vi "CoffeeVending.vi"() -> ()   [LabVIEW 2020, in "CoffeeVending.lvlib"]
uses:
  CoffeeVending.lvlib
  TypeDef/QOperation.ctl
  TypeDef/CoffeeVendingCluster.ctl
  <vilib>/Utility/config.llb/Config Data RefNum.ctl
  <vilib>/Utility/config.llb/Read Key (I32).vi
  <vilib>/Utility/config.llb/Read Key (Boolean).vi
  <vilib>/Utility/config.llb/NI_LVConfig.lvlib
panel:
  in  "Power":bool
  out "Total Cups":i32
  out "Elapsed Time":i32
  out "Dispensing":bool
  out "Brewing":bool
  out "Grinding":bool
  out "Heating":bool
  out "Purging":bool
  out "Low Milk":bool
  out "Low Bean":bool
  out "Low Water":bool
  out "Dispenser":dbl(slide) scale=0.0..60.0
  out "Chamber":dbl(slide) scale=0.0..60.0
  in  "Milk Level":dbl(slide) scale=0.0..100.0
  in  "Bean Level":dbl(slide) scale=0.0..100.0
  in  "Water Level":dbl(slide) scale=0.0..100.0
  in  "Vending Type":i32(knob) scale=0.0..2.0
  in  "Carafe":bool
  in  "Cup":bool
  in  "error in":errorcluster
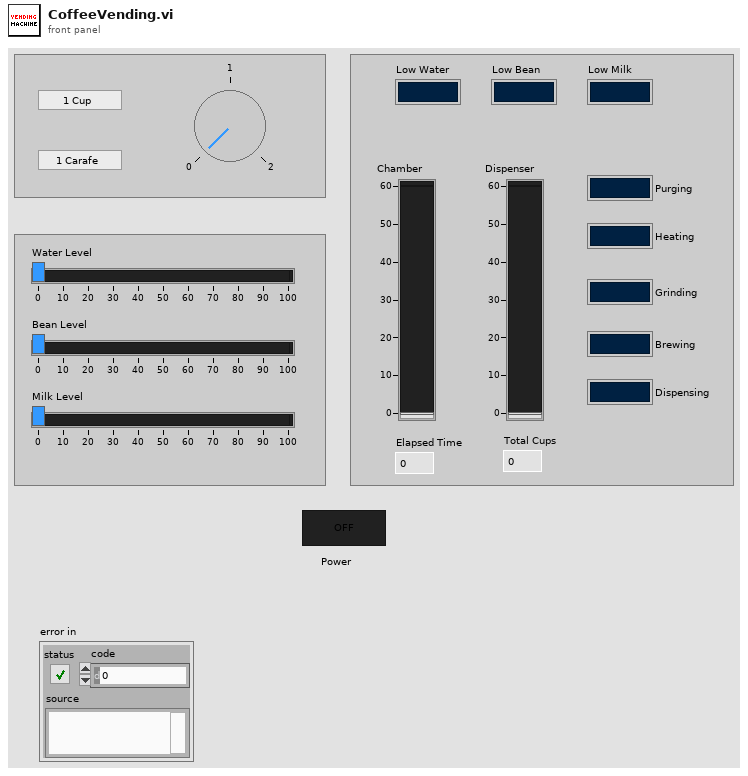
[diagram p1: front panel]
types:
  T1 = typedef "CoffeeVending.lvlib/CoffeeVendingCluster.ctl" = cluster{"Carafe":bool, "Cup":bool, "Water Level":dbl, "Bean Level":dbl, "Milk Level":dbl, "Low Milk":bool, "Low Bean":bool, "Low Water":bool, "Dispenser":dbl, "Chamber":dbl, "Purging":bool, "Brewing":bool, "Heating":bool, "Grinding":bool, "Dispensing":bool, "Elapsed Time":i32, "Total Cups":i32, "File Path":path, "File Reference":T2, "Power":bool, "Start Time":dbl, "Duration":dbl, "Sequence":string[], "Index":i32, "Flag":i32, "Latte":bool}
  T2 = typedef "NI_LVConfig.lvlib/Config Data RefNum.ctl" = refnum<k1>
  T3 = typedef "CoffeeVending.lvlib/QOperation.ctl" = enum16{"Init", "Enqueue", "Dequeue", "Enqueue N", "Enstack", "Release", "Flush"}
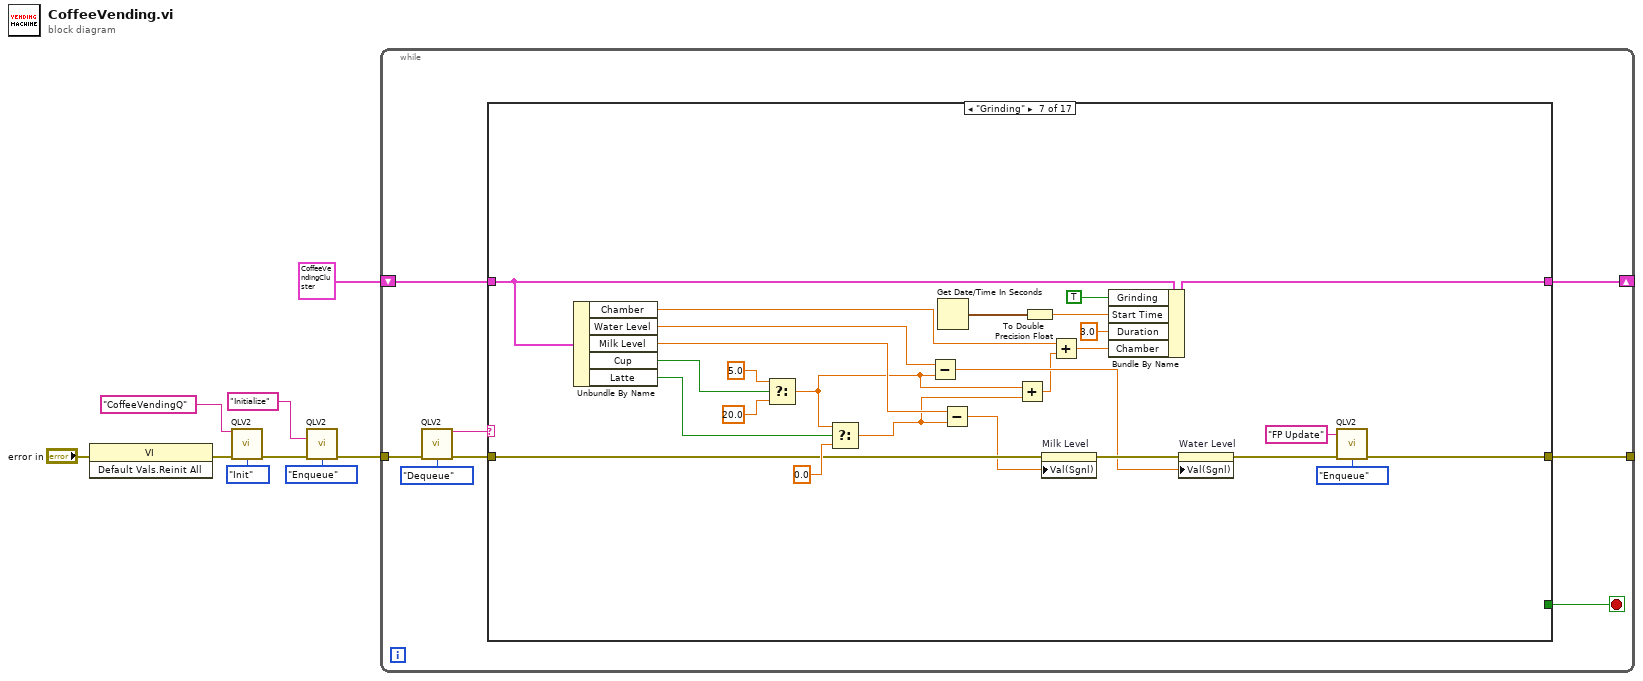
[diagram p0: block diagram]
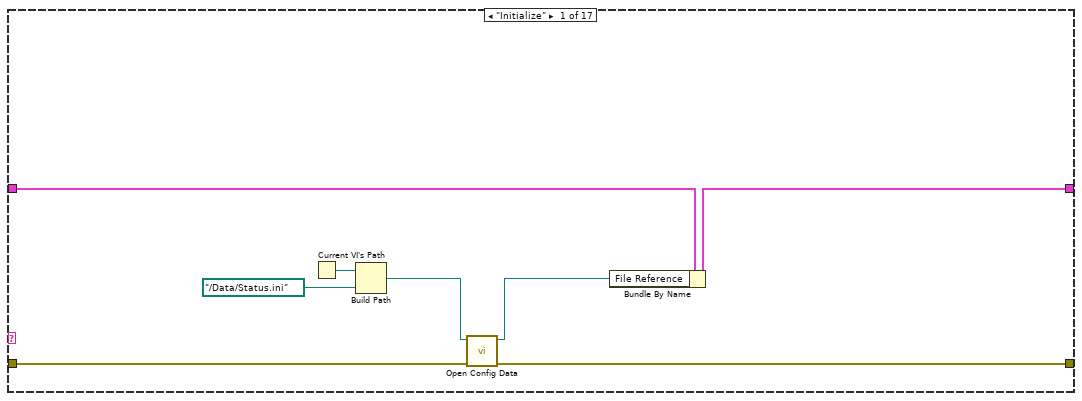
[diagram p2: hidden frame]
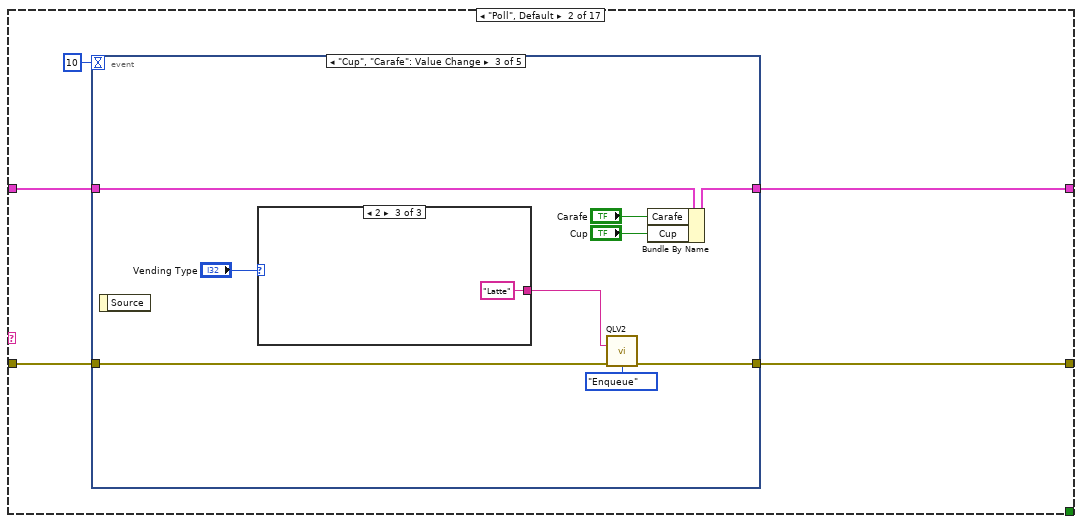
[diagram p3: hidden frame]
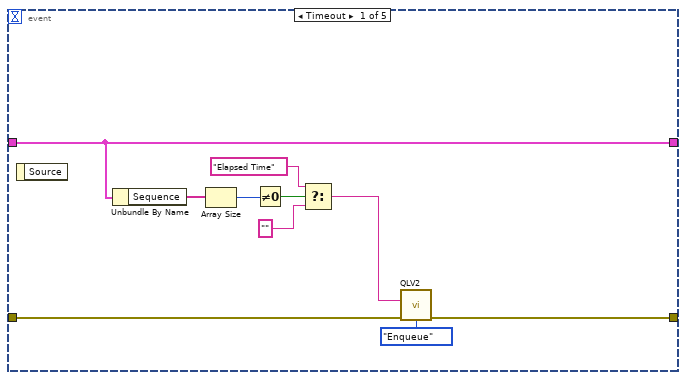
[diagram p4: hidden frame]
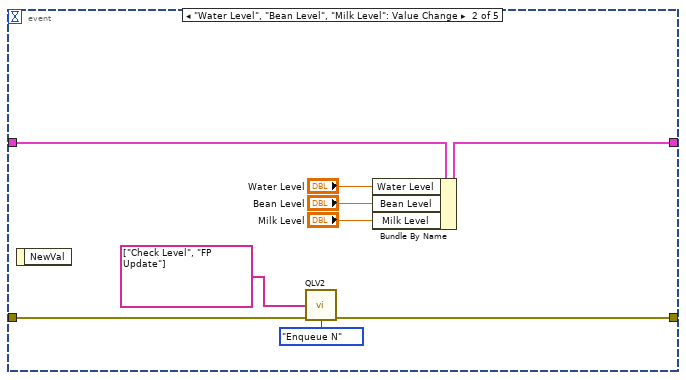
[diagram p5: hidden frame]
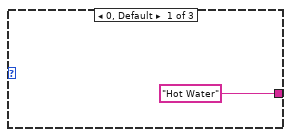
[diagram p6: hidden frame]
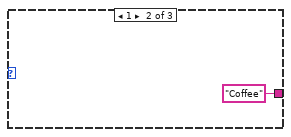
[diagram p7: hidden frame]
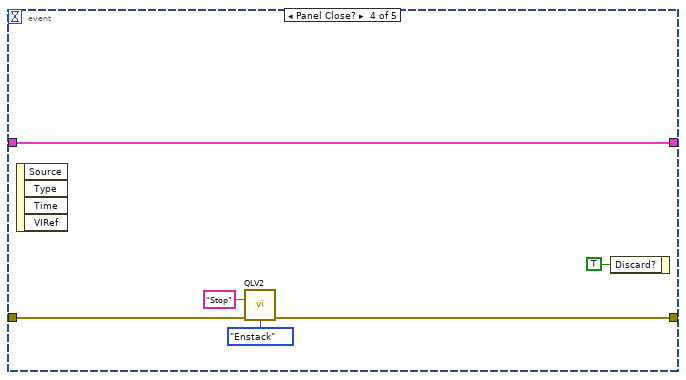
[diagram p8: hidden frame]
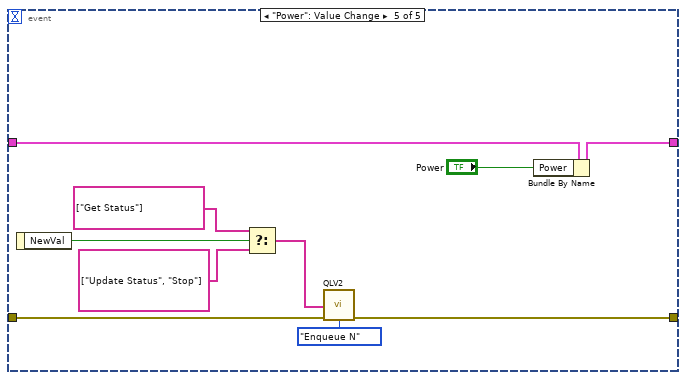
[diagram p9: hidden frame]
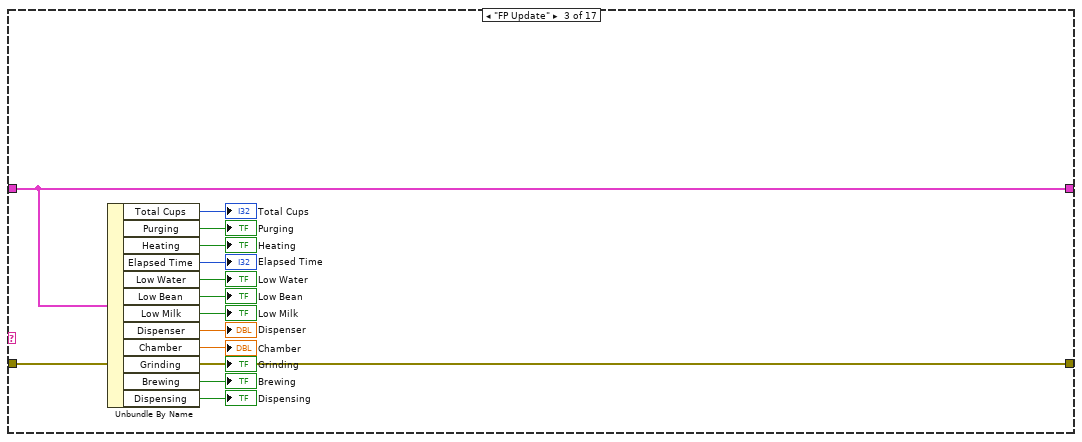
[diagram p10: hidden frame]
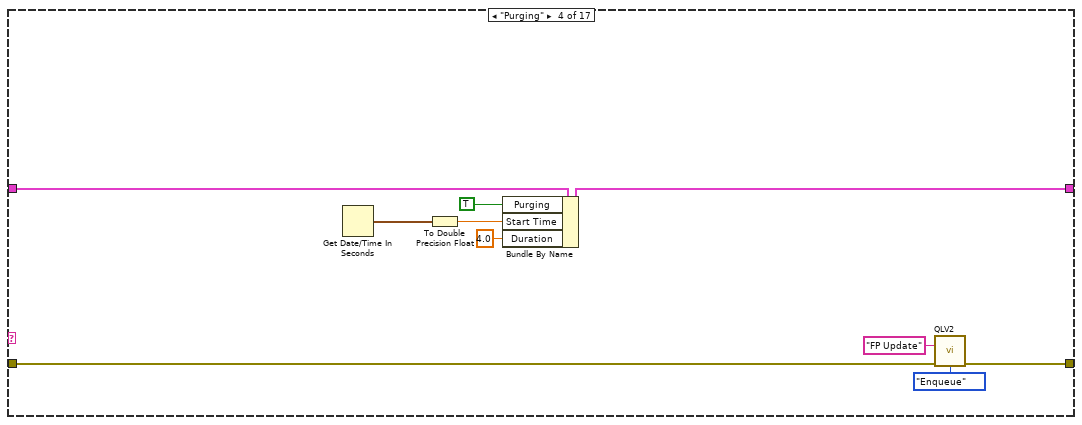
[diagram p11: hidden frame]
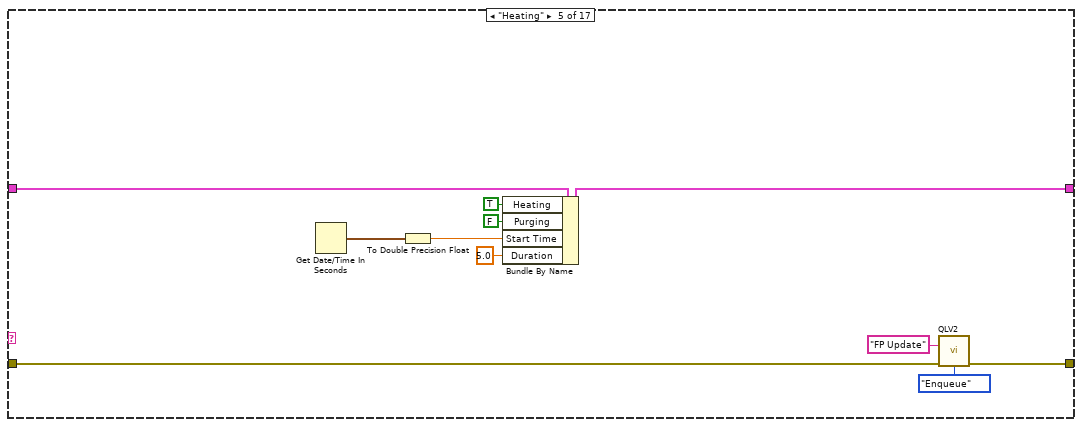
[diagram p12: hidden frame]
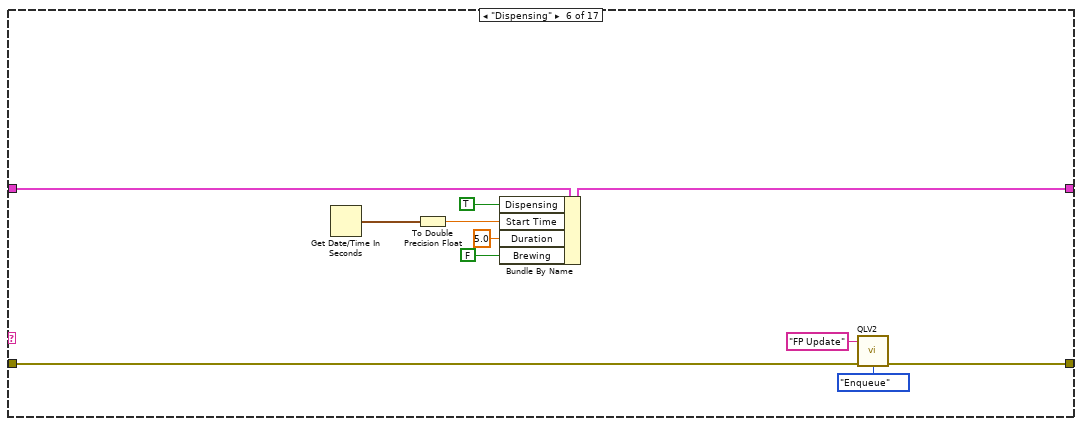
[diagram p13: hidden frame]
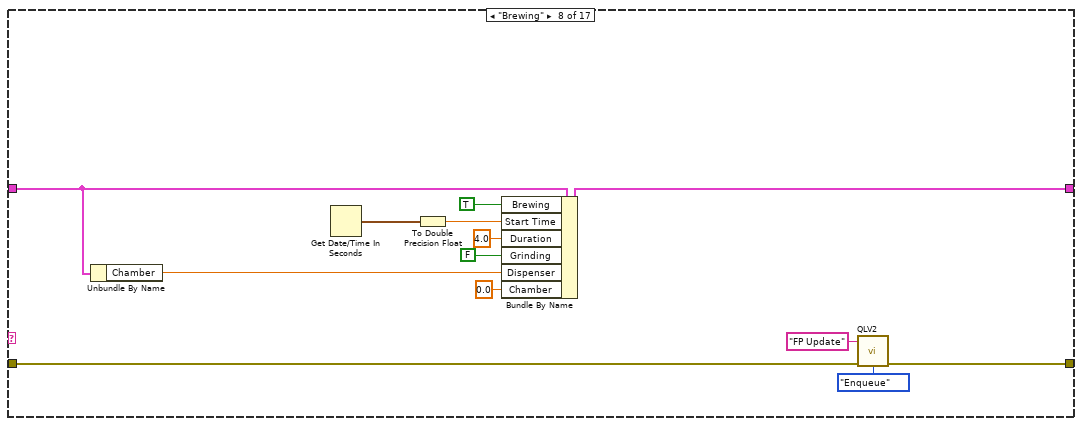
[diagram p14: hidden frame]
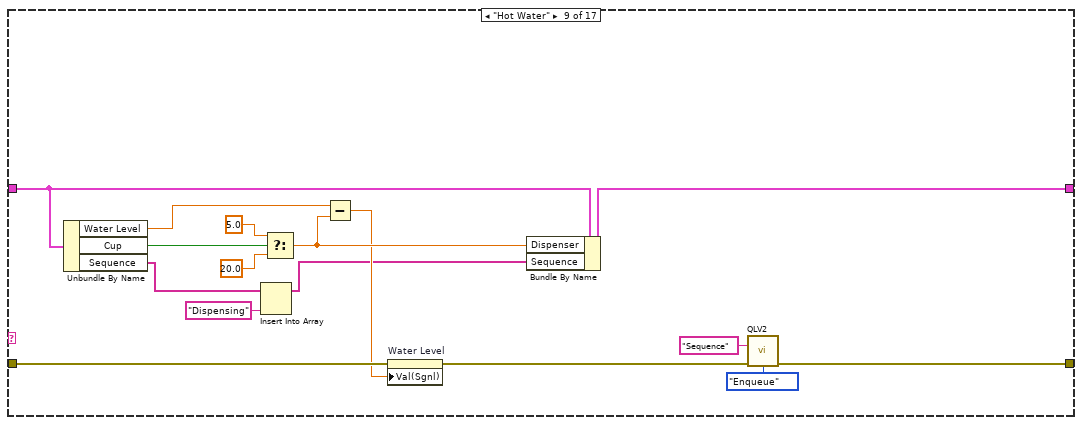
[diagram p15: hidden frame]
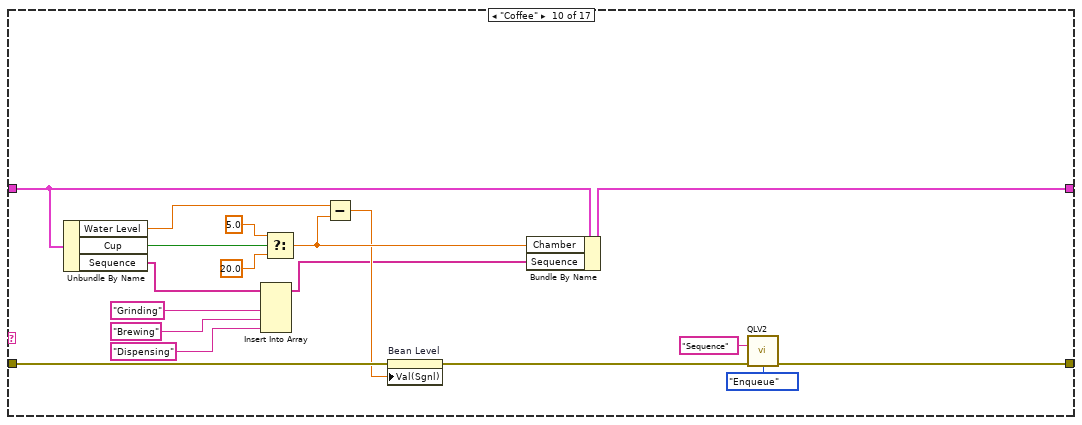
[diagram p16: hidden frame]
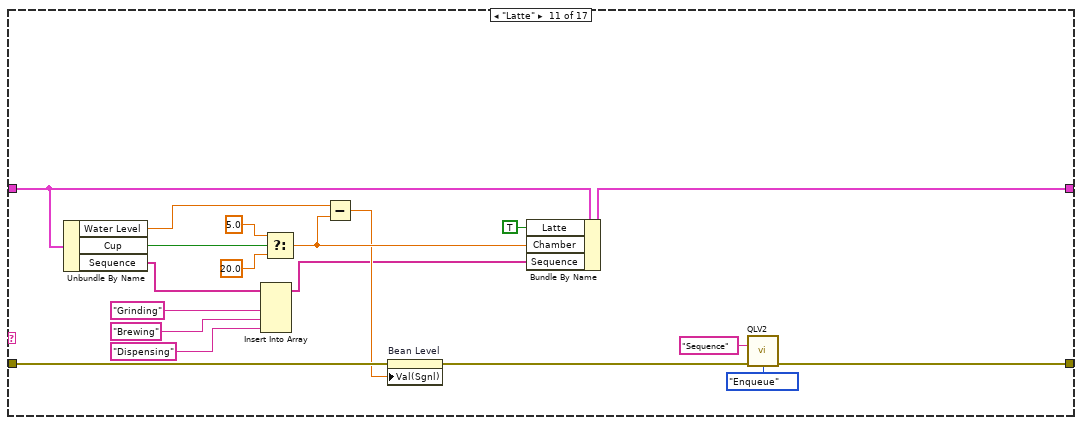
[diagram p17: hidden frame]
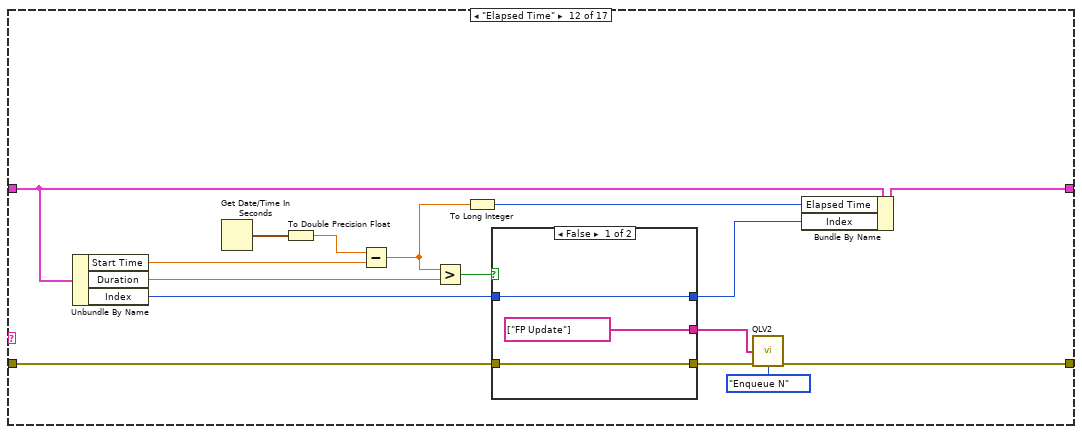
[diagram p18: hidden frame]
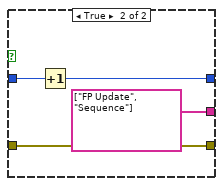
[diagram p19: hidden frame]
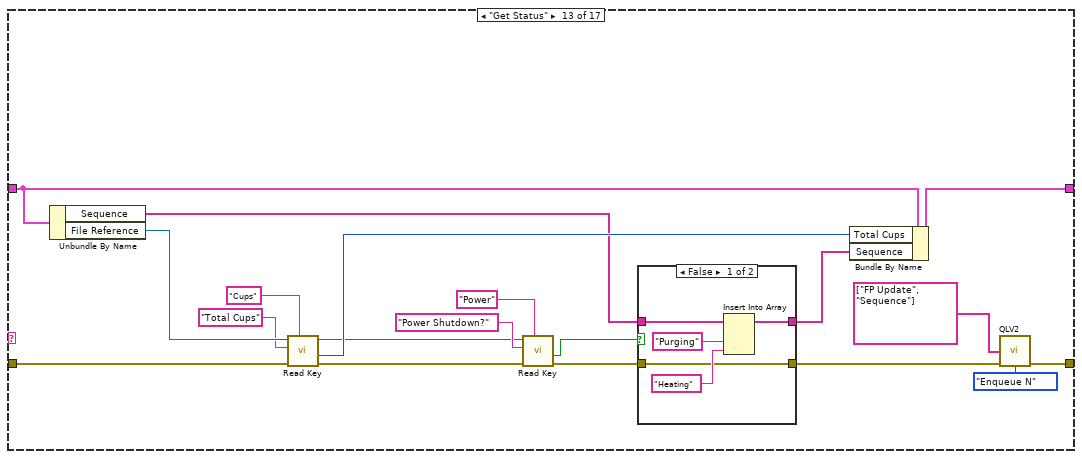
[diagram p20: hidden frame]
diagram:
  n1 = invoke class="VI" method="Default Vals.Reinit All"(error in="error in") -> (error out=w8:errorcluster)  [unwired: 2 in, 2 out]
  n2 = call "QLV2.vi"("Name"="CoffeeVendingQ", "error in"=w8, "Operation"=QOperation."Init") -> ("error out"=w5:errorcluster)  [unwired: 11 in, 1 out]
  n3 = call "QLV2.vi"("States"="Initialize", "error in"=w5, "Operation"=QOperation."Enqueue") -> ("error out"=w2:errorcluster)  [unwired: 11 in, 1 out]
  n4 = while {
    tunnel: w2 -> [w17]
    shift-right: [w12] -> _
    shift-left: T1 {"Carafe"=FALSE, "Cup"=FALSE, "Water Level"=0.0, "Bean Level"=0.0, "Milk Level"=0.0, "Low Milk"=FALSE, "Low Bean"=FALSE, "Low Water"=FALSE, "Dispenser"=0.0, "Chamber"=0.0, "Purging"=FALSE, "Brewing"=FALSE, "Heating"=FALSE, "Grinding"=FALSE, "Dispensing"=FALSE, "Elapsed Time"=0, "Total Cups"=0, "File Path"=path "", "File Reference"=refnum, "Power"=FALSE, "Start Time"=0.0, "Duration"=0.0, "Sequence"=[], "Index"=0, "Flag"=0, "Latte"=FALSE} -> [w13]
    tunnel: [w11] -> _
    stop <- w10 stop-if-true
    n5 = call "QLV2.vi"("error in"=w17, "Operation"=QOperation."Dequeue") -> ("State Out"=w15:string, "error out"=w14:errorcluster)  [unwired: 12 in]
    n6 = case shown="\"Grinding\"" w15 {
      tunnel: w14 -> [w18 w27 w89 w97 w106 w115 w132 w155 w173 w191 w210 w217 w256 w273 w308 w313 w326]
      tunnel: w13 -> [w25 w29 w90 w101 w112 w123 w141 w152 w175 w193 w212 w228 w251 w275 w303 w318 w329]
      tunnel: [w24 w28 w90 w100 w111 w122 w149 w162 w174 w192 w211 w227 w250 w274 w312 w317 w329] -> w12
      tunnel: [w21 w26 w89 w96 w105 w114 w142 w154 w164 w182 w201 w224 w248 w280 w307 w313 w323] -> w11
      tunnel: [_ _ _ _ _ _ _ _ _ _ _ _ _ _ _ _ TRUE] -> w10
      frame "Initialize" {
        n7 = Current VI's Path() -> (path=w23:path)
        n8 = Build Path(base path=w23, name or relative path=path "../Data/Status.ini") -> (appended path=w20:path)
        n9 = call <vilib>:"Open Config Data.vi"("error in (no error)"=w18, "configuration file path"=w20) -> ("error out"=w21:errorcluster, "refnum"=w19:T2)  [unwired: 7 in, 1 out]
        n10 = Bundle By Name(cluster=w25, "File Reference"=w19) -> (w24:T1)
      }
      frame "Poll", Default {
        n11 = event shown="[2] \"Cup\", \"Carafe\": Value Change" {
          selector: _ -> [_ _ _ _ _]
          dyn-events: _ -> [_ _ _ _ _]
          timeout: 10 -> [_ _ _ _ _]
          tunnel: w29 -> [w40 w49 w54 w62 w73]
          tunnel: [w40 w48 w52 w62 w72] -> w28
          tunnel: w27 -> [w33 w46 w56 w65 w76]
          tunnel: [w32 w45 w55 w64 w75] -> w26
          event Timeout {
            n12 = event-data() -> ()  [unwired: 1 in, 1 out]
            n13 = Unbundle By Name(w40) -> ("Sequence"=w39:string[])
            n14 = Array Size(array=w39) -> (size(s)=w38:i32)
            n15 = Not Equal To 0?(x=w38) -> (x != 0?=w37:bool)
            n16 = Select(t="Elapsed Time", s=w37, f="") -> (s? t:f=w31:string)
            n17 = call "QLV2.vi"("States"=w31, "error in"=w33, "Operation"=QOperation."Enqueue") -> ("error out"=w32:errorcluster)  [unwired: 11 in, 1 out]
          }
          event "Water Level", "Bean Level", "Milk Level": Value Change {
            n18 = event-data() -> ()  [unwired: 1 in, 1 out]
            n19 = call "QLV2.vi"("States[]"=string[] ["Check Level", "FP Update"], "error in"=w46, "Operation"=QOperation."Enqueue N") -> ("error out"=w45:errorcluster)  [unwired: 11 in, 1 out]
            n20 = Bundle By Name(cluster=w49, "Water Level"="Water Level", "Bean Level"="Bean Level", "Milk Level"="Milk Level") -> (w48:T1)
          }
          event "Cup", "Carafe": Value Change {
            n21 = event-data() -> ()  [unwired: 1 in, 1 out]
            n22 = case shown="2" "Vending Type" {
              tunnel: ["Hot Water" ("State Out") "Coffee" ("State Out") "Latte" ("State Out")] -> w53
              frame 0, Default {
              }
              frame 1 {
              }
              frame 2 {
              }
            }
            n23 = call "QLV2.vi"("States"=w53, "error in"=w56, "Operation"=QOperation."Enqueue") -> ("error out"=w55:errorcluster)  [unwired: 11 in, 1 out]
            n24 = Bundle By Name(cluster=w54, "Carafe"="Carafe", "Cup"="Cup") -> (w52:T1)
          }
          event Panel Close? {
            n25 = event-data() -> ()  [unwired: 1 in, 4 out]
            n26 = call "QLV2.vi"("States"="Stop", "error in"=w65, "Operation"=QOperation."Enstack") -> ("error out"=w64:errorcluster)  [unwired: 11 in, 1 out]
            n27 = event-data("Discard?"=TRUE) -> ()  [unwired: 1 in, 1 out]
          }
          event "Power": Value Change {
            n28 = event-data() -> ("NewVal"=w74:bool)  [unwired: 1 in]
            n29 = Select(t=string[] ["Get Status"] ("States[]"), s=w74, f=string[] ["Update Status", "Stop"] ("States[]")) -> (s? t:f=w70:string[])
            n30 = call "QLV2.vi"("States[]"=w70, "error in"=w76, "Operation"=QOperation."Enqueue N") -> ("error out"=w75:errorcluster)  [unwired: 11 in, 1 out]
            n31 = Bundle By Name(cluster=w73, "Power"="Power") -> (w72:T1)
          }
        }
      }
      frame "FP Update" {
        n32 = Unbundle By Name(w90) -> ("Total Cups"=→"Total Cups":i32, "Purging"=→"Purging":bool, "Heating"=→"Heating":bool, "Elapsed Time"=→"Elapsed Time":i32, "Low Water"=→"Low Water":bool, "Low Bean"=→"Low Bean":bool, "Low Milk"=→"Low Milk":bool, "Dispenser"=→"Dispenser":dbl, "Chamber"=→"Chamber":dbl, "Grinding"=→"Grinding":bool, "Brewing"=→"Brewing":bool, "Dispensing"=→"Dispensing":bool)
      }
      frame "Purging" {
        n33 = Get Date/Time In Seconds() -> (seconds since 1Jan1904=w94:timestamp)
        n34 = To Double Precision Float(number=w94) -> (double precision float=w93:dbl)
        n35 = Bundle By Name(cluster=w101, "Purging"=TRUE, "Start Time"=w93, "Duration"=4.0) -> (w100:T1)
        n36 = call "QLV2.vi"("States"="FP Update", "error in"=w97, "Operation"=QOperation."Enqueue") -> ("error out"=w96:errorcluster)  [unwired: 11 in, 1 out]
      }
      frame "Heating" {
        n37 = Get Date/Time In Seconds() -> (seconds since 1Jan1904=w104:timestamp)
        n38 = To Double Precision Float(number=w104) -> (double precision float=w103:dbl)
        n39 = Bundle By Name(cluster=w112, "Heating"=TRUE, "Purging"=FALSE, "Start Time"=w103, "Duration"=5.0) -> (w111:T1)
        n40 = call "QLV2.vi"("States"="FP Update", "error in"=w106, "Operation"=QOperation."Enqueue") -> ("error out"=w105:errorcluster)  [unwired: 11 in, 1 out]
      }
      frame "Dispensing" {
        n41 = Get Date/Time In Seconds() -> (seconds since 1Jan1904=w120:timestamp)
        n42 = To Double Precision Float(number=w120) -> (double precision float=w119:dbl)
        n43 = Bundle By Name(cluster=w123, "Dispensing"=TRUE, "Start Time"=w119, "Duration"=5.0, "Brewing"=FALSE) -> (w122:T1)
        n44 = call "QLV2.vi"("States"="FP Update", "error in"=w115, "Operation"=QOperation."Enqueue") -> ("error out"=w114:errorcluster)  [unwired: 11 in, 1 out]
      }
      frame "Grinding" {
        n45 = Unbundle By Name(w141) -> ("Chamber"=w126:dbl, "Water Level"=w134:dbl, "Milk Level"=w133:dbl, "Cup"=w138:bool, "Latte"=w136:bool)
        n46 = Select(t=5.0, s=w138, f=20.0) -> (s? t:f=w128:dbl)
        n47 = Select(t=w128, s=w136, f=0.0) -> (s? t:f=w127:dbl)
        n48 = Subtract(x=w134, y=w128) -> (x-y=w130:dbl)
        n49 = Get Date/Time In Seconds() -> (seconds since 1Jan1904=w147:timestamp)
        n50 = Subtract(x=w133, y=w127) -> (x-y=w129:dbl)
        n51 = Add(x=w128, y=w127) -> (x+y=w125:dbl)
        n52 = To Double Precision Float(number=w147) -> (double precision float=w146:dbl)
        n53 = property on="Milk Level" class="Slide (strict)"(error in=w132, "Val(Sgnl)"=w129) -> (error out=w131:errorcluster)  [unwired: 1 in, 1 out]
        n54 = Add(x=w126, y=w125) -> (x+y=w124:dbl)
        n55 = Bundle By Name(cluster=w141, "Grinding"=TRUE ("Dispensing"), "Start Time"=w146, "Duration"=3.0, "Chamber"=w124) -> (w149:T1)
        n56 = property on="Water Level" class="Slide (strict)"(error in=w131, "Val(Sgnl)"=w130) -> (error out=w137:errorcluster)  [unwired: 1 in, 1 out]
        n57 = call "QLV2.vi"("States"="FP Update", "error in"=w137, "Operation"=QOperation."Enqueue") -> ("error out"=w142:errorcluster)  [unwired: 11 in, 1 out]
      }
      frame "Brewing" {
        n58 = Unbundle By Name(w152) -> ("Chamber"=w151:dbl)
        n59 = Get Date/Time In Seconds() -> (seconds since 1Jan1904=w160:timestamp)
        n60 = To Double Precision Float(number=w160) -> (double precision float=w159:dbl)
        n61 = Bundle By Name(cluster=w152, "Brewing"=TRUE ("Dispensing"), "Start Time"=w159, "Duration"=4.0, "Grinding"=FALSE, "Dispenser"=w151, "Chamber"=0.0) -> (w162:T1)
        n62 = call "QLV2.vi"("States"="FP Update", "error in"=w155, "Operation"=QOperation."Enqueue") -> ("error out"=w154:errorcluster)  [unwired: 11 in, 1 out]
      }
      frame "Hot Water" {
        n63 = Unbundle By Name(w175) -> ("Water Level"=w172:dbl, "Cup"=w178:bool, "Sequence"=w169:string[])
        n64 = Insert Into Array(array=w169, new element="Dispensing" ("new element/subarray")) -> (w167:string[])  [unwired: 1 in]
        n65 = Select(t=5.0, s=w178, f=20.0) -> (s? t:f=w171:dbl)
        n66 = Subtract(x=w172, y=w171) -> (x-y=w170:dbl)
        n67 = property on="Water Level" class="Slide (strict)"(error in=w173, "Val(Sgnl)"=w170) -> (error out=w165:errorcluster)  [unwired: 1 in, 1 out]
        n68 = Bundle By Name(cluster=w175, "Dispenser"=w171, "Sequence"=w167) -> (w174:T1)
        n69 = call "QLV2.vi"("States"="Sequence", "error in"=w165, "Operation"=QOperation."Enqueue") -> ("error out"=w164:errorcluster)  [unwired: 11 in, 1 out]
      }
      frame "Coffee" {
        n70 = Unbundle By Name(w193) -> ("Water Level"=w190:dbl, "Cup"=w196:bool, "Sequence"=w187:string[])
        n71 = Insert Into Array(array=w187, new element #1="Grinding" ("new element/subarray"), new element #2="Brewing" ("new element/subarray"), new element #3="Dispensing" ("new element/subarray")) -> (w185:string[])  [unwired: 1 in]
        n72 = Select(t=5.0, s=w196, f=20.0) -> (s? t:f=w189:dbl)
        n73 = Subtract(x=w190, y=w189) -> (x-y=w188:dbl)
        n74 = property on="Bean Level" class="Slide (strict)"(error in=w191, "Val(Sgnl)"=w188) -> (error out=w183:errorcluster)  [unwired: 1 in, 1 out]
        n75 = Bundle By Name(cluster=w193, "Chamber"=w189, "Sequence"=w185) -> (w192:T1)
        n76 = call "QLV2.vi"("States"="Sequence", "error in"=w183, "Operation"=QOperation."Enqueue") -> ("error out"=w182:errorcluster)  [unwired: 11 in, 1 out]
      }
      frame "Latte" {
        n77 = Unbundle By Name(w212) -> ("Water Level"=w209:dbl, "Cup"=w215:bool, "Sequence"=w206:string[])
        n78 = Insert Into Array(array=w206, new element #1="Grinding" ("new element/subarray"), new element #2="Brewing" ("new element/subarray"), new element #3="Dispensing" ("new element/subarray")) -> (w204:string[])  [unwired: 1 in]
        n79 = Select(t=5.0, s=w215, f=20.0) -> (s? t:f=w208:dbl)
        n80 = Subtract(x=w209, y=w208) -> (x-y=w207:dbl)
        n81 = property on="Bean Level" class="Slide (strict)"(error in=w210, "Val(Sgnl)"=w207) -> (error out=w202:errorcluster)  [unwired: 1 in, 1 out]
        n82 = Bundle By Name(cluster=w212, "Latte"=TRUE, "Chamber"=w208, "Sequence"=w204) -> (w211:T1)
        n83 = call "QLV2.vi"("States"="Sequence", "error in"=w202, "Operation"=QOperation."Enqueue") -> ("error out"=w201:errorcluster)  [unwired: 11 in, 1 out]
      }
      frame "Elapsed Time" {
        n84 = Unbundle By Name(w228) -> ("Start Time"=w230:dbl, "Duration"=w223:dbl, "Index"=w220:i32)
        n85 = Get Date/Time In Seconds() -> (seconds since 1Jan1904=w231:timestamp)
        n86 = To Double Precision Float(number=w231) -> (double precision float=w229:dbl)
        n87 = Subtract(x=w229, y=w230) -> (x-y=w222:dbl)
        n88 = Greater?(x=w222, y=w223) -> (0:w221:bool)
        n89 = To Long Integer(number=w222) -> (32bit integer=w226:i32)
        n90 = case shown="False" w221 {
          tunnel: w220 -> [w234 w238]
          tunnel: [w234 w237] -> w219
          tunnel: [string[] ["FP Update"] ("States[]") string[] ["FP Update", "Sequence"] ("States[]")] -> w218
          tunnel: [w232 w235] -> w216
          tunnel: w217 -> [w232 w235]
          frame False {
          }
          frame True {
            n91 = Increment(x=w238) -> (x+1=w237:i32)
          }
        }
        n92 = call "QLV2.vi"("States[]"=w218, "error in"=w216, "Operation"=QOperation."Enqueue N") -> ("error out"=w224:errorcluster)  [unwired: 11 in, 1 out]
        n93 = Bundle By Name(cluster=w228, "Elapsed Time"=w226, "Index"=w219) -> (w227:T1)
      }
      frame "Get Status" {
        n94 = Unbundle By Name(w251) -> ("Sequence"=w241:string[], "File Reference"=w257:T2)
        n95 = call-poly <vilib>:"Read Key.vi"("section"="Cups", "error in (no error)"=w256, "key"="Total Cups", "refnum"=w257) -> ("error out"=w247:errorcluster, "value"=w249:i32, "refnum out"=w246:T2)  [unwired: 4 in, 1 out]
        n96 = call-poly <vilib>:"Read Key.vi"("section"="Power", "error in (no error)"=w247, "key"="Power Shutdown?", "refnum"=w246) -> ("error out"=w243:errorcluster, "value"=w242:bool)  [unwired: 4 in, 2 out]
        n97 = case shown="False" w242 {
          tunnel: w243 -> [w258 w263]
          tunnel: w241 -> [w261 w266]
          tunnel: [w260 w264] -> w240
          tunnel: [w258 w263] -> w239
          frame False {
            n98 = Insert Into Array(array=w261, new element #1="Purging" ("new element/subarray"), new element #2="Heating" ("new element/subarray")) -> (w260:string[])  [unwired: 1 in]
          }
          frame True {
            n99 = Insert Into Array(array=w266, new element="Heating" ("new element/subarray")) -> (w264:string[])  [unwired: 1 in]
          }
        }
        n100 = Bundle By Name(cluster=w251, "Total Cups"=w249, "Sequence"=w240) -> (w250:T1)
        n101 = call "QLV2.vi"("States[]"=string[] ["FP Update", "Sequence"], "error in"=w239, "Operation"=QOperation."Enqueue N") -> ("error out"=w248:errorcluster)  [unwired: 11 in, 1 out]
      }
      frame "Sequence" {
        n102 = Unbundle By Name(w275) -> ("Elapsed Time"=w268:i32, "Sequence"=w279:string[], "Index"=w276:i32)
        n103 = Array Size(array=w279) -> (size(s)=w278:i32)
        n104 = Greater?(x=w278, y=w276) -> (0:w277:bool)
        n105 = case shown="False" w277 {
          tunnel: w276 -> [_ w288]
          tunnel: ["Process Complete" w291] -> w269
          tunnel: w279 -> [_ w289]
          tunnel: w273 -> [w286 w290]
          tunnel: [w286 w290] -> w272
          tunnel: [string[] [] ("Sequence") w289] -> w271
          tunnel: [0 ("Index") w288] -> w270
          tunnel: w268 -> [_ w287]
          tunnel: [0 ("Elapsed Time") w287] -> w267
          frame False {
          }
          frame True {
            n106 = Index Array(array=w289, index=w288) -> (element=w291:string)
          }
        }
        n107 = Bundle By Name(cluster=w275, "Elapsed Time"=w267, "Sequence"=w271, "Index"=w270) -> (w274:T1)
        n108 = call "QLV2.vi"("States"=w269, "error in"=w272, "Operation"=QOperation."Enqueue") -> ("error out"=w280:errorcluster)  [unwired: 11 in, 1 out]
      }
      frame "Process Complete" {
        n109 = Unbundle By Name(w303) -> ("Total Cups"=w294:i32, "Flag"=w302:i32, "Cup"=w297:bool)
        n110 = Equal To 0?(x=w302) -> (x = 0?=w301:bool)
        n111 = Select(t=1, s=w297, f=4) -> (s? t:f=w293:i32)
        n112 = Subtract(x=w294, y=w293) -> (x-y=w292:i32)
        n113 = Select(t=w294, s=w301, f=w292) -> (s? t:f=w299:i32)
        n114 = Bundle By Name(cluster=w303, "Flag"=1, "Heating"=FALSE, "Purging"=FALSE, "Dispensing"=FALSE, "Dispenser"=0.0, "Chamber"=0.0, "Total Cups"=w299) -> (w312:T1)
        n115 = call "QLV2.vi"("States[]"=string[] ["Check Level", "FP Update"], "error in"=w308, "Operation"=QOperation."Enqueue N") -> ("error out"=w307:errorcluster)  [unwired: 11 in, 1 out]
      }
      frame "Check Level" {
        w319 = 30.0 ("y")
        n116 = Unbundle By Name(w318) -> ("Water Level"=w322:dbl, "Bean Level"=w321:dbl, "Milk Level"=w320:dbl)
        n117 = Less?(x=w322, y=w319) -> (x < y?=w316:bool)
        n118 = Less?(x=w320, y=w319) -> (x < y?=w314:bool)
        n119 = Less?(x=w321, y=w319) -> (x < y?=w315:bool)
        n120 = Bundle By Name(cluster=w318, "Low Water"=w316, "Low Bean"=w315, "Low Milk"=w314) -> (w317:T1)
      }
      frame "Stop" {
        n121 = call "QLV2.vi"("error in"=w326, "Operation"=QOperation."Flush") -> ("error out"=w324:errorcluster)  [unwired: 12 in, 1 out]
        n122 = call "QLV2.vi"("error in"=w324, "Operation"=QOperation."Release") -> ("error out"=w323:errorcluster)  [unwired: 12 in, 1 out]
      }
    }
  }
